vi "DB Import Action - Create Chans.vi"(8 "error in (no error)":errorcluster, 10 "selected path":path, 11 "Node Ptr":u64) -> (0 "error out":errorcluster, 2 "selected path out":path caption="selected path", 3 "Node Ptr dup":u64)   [LabVIEW 2019, in "Ballard Arinc-429 System Explorer.lvlib"]
uses:
  Ballard Arinc-429 System Explorer.lvlib
  Create Sysdef Tree Labels.vi
  Build Label Properties.vi
  Shared/Controls and Global/Global.vi
  <vilib>/NI VeriStand/Custom Device Tools/Custom Device Utility Library/NI VeriStand - Search for Item.vi
  <vilib>/NI VeriStand/Custom Device Tools/Custom Device Utility Library/NI VeriStand - Search for Item by GUID.vi
  <vilib>/NI VeriStand/Custom Device API/NI VeriStand - Add Custom Device Section.vi
  <vilib>/NI VeriStand/Custom Device API/NI VeriStand - Add Custom Device Channel.vi
  Create Tx Word Description.vi
  <vilib>/NI VeriStand/Custom Device API/NI VeriStand - Set Item Description.vi
  <vilib>/NI VeriStand/Custom Device API/Custom Device API.lvlib
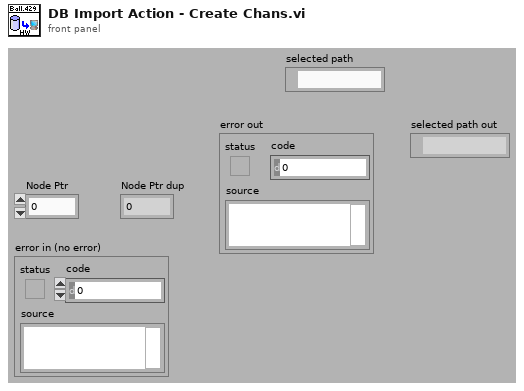
[diagram p1: front panel]
types:
  T1 = typedef "Ballard Arinc-429 System Explorer.lvlib/Ballard_Channel Array.ctl" = T2[]
  T2 = typedef "Ballard Arinc-429 System Explorer.lvlib/Ballard_Channel.ctl" = cluster{"Labels":T3[], "name":string, "number":u8, "direction":T7, "Voltage":dbl, "speed":T8}
  T3 = typedef "Ballard Arinc-429 System Explorer.lvlib/Ballard_Label.ctl" = cluster{"name":string, "xmlName":string, "TxPeriod":u32, "label":u32, "TxRate":dbl, "SDI_Enabled":bool, "SDIValue":u8, "Word":T4, "TransferType":T6, "scheduleBuildUnit":i32, "Initial Enable State":bool}
  T4 = typedef "Ballard Arinc-429 System Explorer.lvlib/Ballard_Word.ctl" = cluster{"InitalValue":u32, "Params":T5[]}
  T5 = typedef "Ballard Arinc-429 System Explorer.lvlib/ARINCParam.ctl" = cluster{"name":string, "startBit":i32, "numberBits":i32, "scaleFactor":dbl, "scaleOffset":dbl, "signed":bool}
  T6 = typedef "Ballard Arinc-429 Shared.lvlib/TransferType.ctl" = enum16{"ScheduledLabel", "Acyclic", "Block", "Strobe"}
  T7 = typedef "Ballard Arinc-429 System Explorer.lvlib/Channel_direction.ctl" = enum16{"429_DIRECTION_RX", "429_DIRECTION_TX"}
  T8 = typedef "Ballard Arinc-429 System Explorer.lvlib/Channel Speed.ctl" = i32
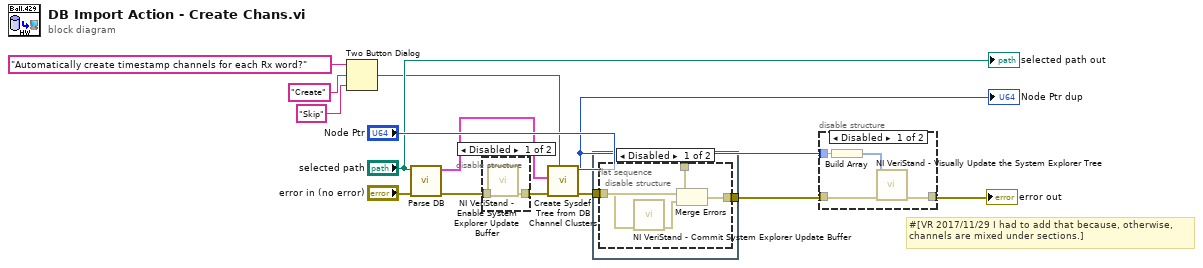
[diagram p0: block diagram]
diagram:
  # "#[VR 2017/11/29 I had to add that because, otherwise,\nchannels are mixed under sections.]"
  n1 = Two Button Dialog(message="Automatically create timestamp channels for each Rx word?", 1:"Skip" ("F button name (\"Cancel\")"), 2:"Create" ("T button name (\"OK\")")) -> (T button?=w6:bool)
  n2 = call "Parse DB.vi"("error in (no error)"="error in (no error)", "Path in"="selected path") -> ("error out"=w1:errorcluster, "channels"=w13:T1)  [unwired: 8 in]
  n3 = disable-structure shown="Disabled" {
    disable-tunnel: [w16 w17] -> w12
    disable-tunnel: w1 -> [w15 w17]
    frame Disabled {
      n4 = call <vilib>:"NI VeriStand - Enable System Explorer Update Buffer.vi"("error in (no error)"=w15) -> ("error out"=w16:errorcluster)  [unwired: 10 in]
    }
    frame Enabled {
    }
  }
  n5 = call "Create Sysdef Tree from DB Channel Clusters.vi"("Autocreate Rx timestamp chans?"=w6, "error in"=w12, "Channels to create"=w13, "Device Ptr"="Node Ptr") -> ("error out"=w10:errorcluster, "Device Ptr dup"=w4:u64)  [unwired: 6 in]
  "Node Ptr dup" <- w4
  n6 = flat-sequence {
    tunnel: w10 -> [w18]
    tunnel: [w19] -> w2
    frame #0 {
      n7 = disable-structure shown="Disabled" {
        disable-tunnel: w18 -> [w23 _]
        disable-tunnel: [w21 w24] -> w19
        disable-tunnel: w18 -> [w20 w24]
        frame Disabled {
          n8 = call <vilib>:"NI VeriStand - Commit System Explorer Update Buffer.vi"("error in (no error)"=w20) -> ("error out"=w22:errorcluster)  [unwired: 10 in]
          n9 = Merge Errors(w23, w22) -> (w21:errorcluster)
        }
        frame Enabled {
        }
      }
    }
  }
  n10 = disable-structure shown="Disabled" {
    disable-tunnel: [w28 w29] -> w5
    disable-tunnel: w4 -> [w27 _]
    disable-tunnel: w2 -> [w25 w29]
    frame Disabled {
      n11 = Build Array(w27) -> (w26:u64[])
      n12 = call "NI VeriStand - Visually Update the System Explorer Tree.vi"("error in (no error)"=w25, "Node IDs"=w26) -> ("error out"=w28:errorcluster)  [unwired: 9 in]
    }
    frame Enabled {
    }
  }
  "error out" <- w5
  "selected path out" <- "selected path"
